vi "Actor Core.vi"(8 "error in":errorcluster, 11 "Nested in":refnum<class "RefNums and UICtrl.lvclass">) -> (0 "error out":errorcluster, 3 "Nested out":refnum<class "Actor.lvclass">)   [LabVIEW 2020, in "RefNums and UICtrl.lvclass"]
doc: "(<B>Filename</B>: Actor Framework.lvlib:Actor.lvclass:Actor Core.vi)\n\nReceives messages to the actor, reacts to them, and initiates any error handling that may shut the actor down.\n\nDescendant classes may override this VI to append parallel tasks for the actor to complete while it handles messages. Overrides use the Call Parent Method node."
uses:
  RefNums and UICtrl.lvclass
  C:/Program Files (x86)/National Instruments/LabVIEW 2020/vi.lib/ActorFramework/Actor/Actor.lvclass
  <vilib>/ActorFramework/Actor/Actor.lvclass
  RefNums and UICtrl.lvclass/RefNums and UICtrl.ctl
  <vilib>/ActorFramework/Actor/Actor.lvclass/Actor.ctl
  <vilib>/ActorFramework/Message Enqueuer/Message Enqueuer.lvclass/Message Enqueuer.ctl
  <vilib>/ActorFramework/Message Enqueuer/Init from Existing Queue.vi
  <vilib>/ActorFramework/Message Enqueuer/Enqueue.vi
  <vilib>/ActorFramework/Stop Msg/Stop Msg.lvclass
  C:/Program Files (x86)/National Instruments/LabVIEW 2020/vi.lib/ActorFramework/Message/Message.lvclass
  <vilib>/ActorFramework/Message Priority Queue/Priority Enqueue.vi
  <vilib>/MGI/Monitored Actor/Monitored Actor/Monitored Actor/Monitored Actor.lvclass
  <vilib>/ActorFramework/Message Enqueuer/Message Enqueuer.lvclass
  C:/Program Files (x86)/National Instruments/LabVIEW 2020/vi.lib/MGI/Monitored Actor/Monitored Actor/Monitored Actor/Monitored Actor.lvclass
  D:/Workspace/LabVIEW/LVToolset/Events for UI Actors/Create Actor from Template/_RefNums and UICtrl/RefNums and UICtrl.lvclass
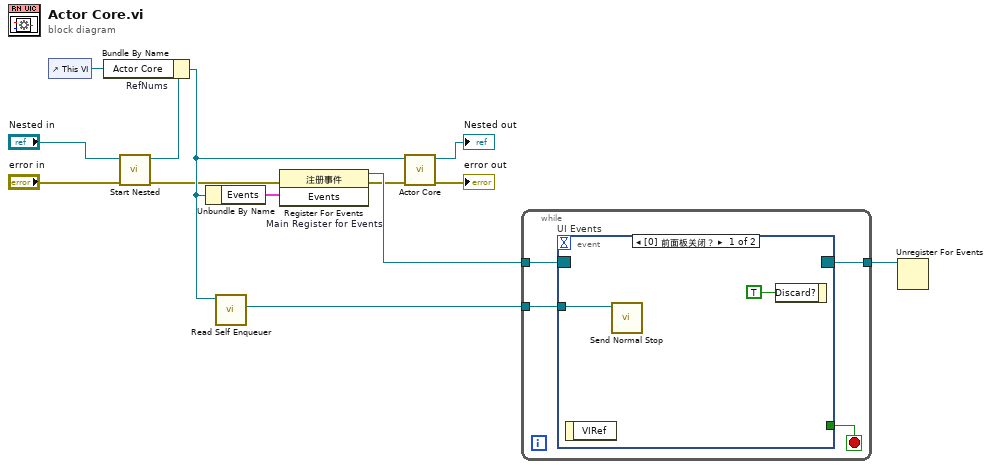
[diagram p0: block diagram]
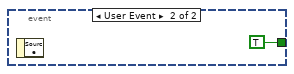
[diagram p2: hidden frame]
diagram:
  n1 = control-ref of="This VI"() -> (w4:refnum<vi>)
  n2 = call "Start Nested.vi"("error in (no error)"="error in", "RefNums and UICtrl 输入"="Nested in") -> ("error out"=w3:errorcluster, "RefNums and UICtrl 输出"=w1:refnum<class "RefNums and UICtrl.lvclass">)  [unwired: 8 in]
  n3 = Bundle By Name "RefNums"(cluster=w1, "Actor Core"=w4) -> (w5:refnum<class "RefNums and UICtrl.lvclass">)
  n4 = Unbundle By Name(w5) -> ("Events"=w10:cluster{"Stop":refnum<user-event>})
  n5 = call <vilib>:"Read Self Enqueuer.vi"("Actor"=w5) -> ("Self Enqueuer"=w8:refnum<class "Message Enqueuer.lvclass">)  [unwired: 10 in]
  n6 = register-events "Main Register for Events"(error in=w3, w10) -> (reference out=w11:refnum<event-registration>, error out=w6:errorcluster)  [unwired: 1 in]
  n7 = call-parent "Actor Core.vi"("error in"=w6, "Actor in"=w5) -> ("error out"=→"error out":errorcluster, "Actor out"=→"Nested out":refnum<class "Actor.lvclass">)  [unwired: 8 in]
  n8 = while {
    tunnel: w11 -> [w17]
    tunnel: [w15] -> w9
    tunnel: w8 -> [w14]
    stop <- w16 stop-if-true
    n9 = event "UI Events" shown="[0] 前面板关闭？" {
      selector: w17 -> [_ _]
      dyn-events: [_ _] -> w15
      timeout: _ -> [_ _]
      tunnel: [_ TRUE] -> w16
      tunnel: w14 -> [w18 _]
      event Panel Close? {
        n10 = event-data() -> ()  [unwired: 1 in, 1 out]
        n11 = call <vilib>:"Send Normal Stop.vi"("Message Enqueuer"=w18) -> ()  [unwired: 10 in, 1 out]
        n12 = event-data("Discard?"=TRUE) -> ()  [unwired: 1 in, 1 out]
      }
      event User Event {
        n13 = event-data() -> ()  [unwired: 1 in, 1 out]
      }
    }
  }
  n14 = Unregister For Events(event registration refnum=w9) -> ()  [unwired: 1 in, 1 out]
